vi "AdjustIfEmpty.vi"(10 "Found":string[](array[string])) -> (2 "FoundAdj":string[](array[string]))   [LabVIEW 2013, in "FindName Task_Manager.lvlib"]
doc: "This VI ensures that the output array is never empty. If the input array IS NOT empty, it is passed to the output untouched. If the input array IS empty, a persistant, very random string is passed as the single element of the output array. The random string is only generated once."
uses:
  FindName Task_Manager.lvlib
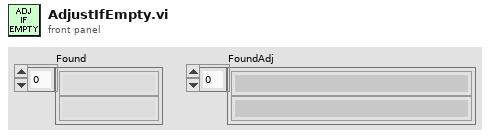
[diagram p1: front panel]
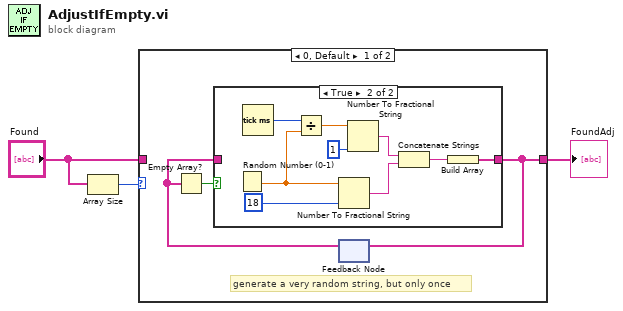
[diagram p0: block diagram]
diagram:
  n1 = Array Size(array="Found") -> (size(s)=w2:i32)
  n2 = case shown="0, Default" w2 {
    tunnel: "Found" -> [_ w17]
    tunnel: [w6 w17] -> w1
    frame 0, Default {
      # "generate a very random string, but only once"
      n3 = feedback #1() -> (w4:string[])  [unwired: 1 in]
      n4 = Empty Array?(array=w4) -> (empty?=w5:bool)
      n5 = case shown="True" w5 {
        tunnel: [w7 w8] -> w6
        tunnel: w4 -> [w7 _]
        frame False {
        }
        frame True {
          n6 = Random Number (0-1)() -> (number: 0 to 1=w9:dbl)
          n7 = Tick Count (ms)() -> (millisecond timer value=w10:u32)
          n8 = Divide(x=w10, y=w9) -> (x/y=w11:dbl)
          n9 = Number To Fractional String(number=w9, precision (6)=i16 18) -> (F-format string=w14:string)  [unwired: 2 in]
          n10 = Number To Fractional String(number=w11, precision (6)=i16 1) -> (F-format string=w15:string)  [unwired: 2 in]
          n11 = Concatenate Strings(w15, w14) -> (w13:string)
          n12 = Build Array(w13) -> (w8:string[])
        }
      }
      n13 = feedback-in #1(w6) -> ()
    }
    frame 1.. {
    }
  }
  "FoundAdj" <- w1
